vi "HexDAQ.vi"() -> ()   [LabVIEW 2020]
doc: "This is the main VI for the HexDAQ project. Contains the front panel controls steers the entire data taking, logging and display."
uses:
  input_params.ctl
  refs_front_panel.ctl
  <extravilib>/ChannelInstances/Tag-a[.](c(a[.](stamp),a[.](dbl)))/Read With Abort.vi
  <extravilib>/ChannelInstances/Tag-bool/Read With Abort.vi
  <extravilib>/ChannelInstances/Tag-t'input_params.ctl'/Write With Abort.vi
  <extravilib>/ChannelInstances/Tag-str/Write With Abort.vi
  <extravilib>/ChannelInstances/Tag-bool/Write With Abort.vi
  <extravilib>/ChannelInstances/Tag-t'data_env.ctl'/Instantiate.vi
  <extravilib>/ChannelInstances/Tag-t'input_params.ctl'/Instantiate.vi
  <extravilib>/ChannelInstances/Tag-str/Instantiate.vi
  <extravilib>/ChannelInstances/Tag-a[.](c(a[.](stamp),a[.](dbl)))/Instantiate.vi
  <extravilib>/ChannelInstances/Tag-bool/Instantiate.vi
  <extravilib>/ChannelInstances/Tag-a[.](c(a[.](stamp),a[.](dbl)))/EndpointRead.vi
  <extravilib>/ChannelInstances/Tag-bool/EndpointRead.vi
  <extravilib>/ChannelInstances/Tag-t'input_params.ctl'/Endpoint.vi
  <extravilib>/ChannelInstances/Tag-str/Endpoint.vi
  <extravilib>/ChannelInstances/Tag-bool/Endpoint.vi
  <extravilib>/ChannelInstances/Tag-bool.lvlib
  <extravilib>/ChannelInstances/Tag-a[.](c(a[.](stamp),a[.](dbl))).lvlib
  <extravilib>/ChannelInstances/Tag-str.lvlib
  user32.dll
  <extravilib>/ChannelInstances/Tag-t'input_params.ctl'.lvlib
panel:
  in  "Annealing (min)":string
  in  "Fluence (neq)":string
  in  "Temperature (deg C)":string
  in  "Measure\nevery n-th*":dbl=1.0
  out "Switchboard enable":bool=TRUE
  in  "HexPlot binary path":path=path "C:/Users/calice/Desktop/ProbeStation/HGCAL_sensor_tests-CALICE_6in_256ch/bin/HexPlot.exe"
  in  "Source device":T1(ring)=enum."Source_6487"
  in  "LCR device":enum16{"LCR_E4980", "AGILENT_4263X"}(ring)
  in  "Mask pad above (uA)":dbl=5.0
  in  "Mask pads":string
  in  "Source interlock?":bool=TRUE
  out "Missing current [%]\n(Sum cells - tot)/tot":dbl format="%#.0f"
  in  "Abort 3":bool
  in  "Polarity: switch only affects contact test":enum32{"Radio Selection 1", "Radio Selection 2"}(radio)
  in  "CV Switch Delay (s)":dbl=0.3
  in  "IV Switch Delay (s)":dbl=0.3
  in  "CV voltage file":path=path "C:/Users/calice/Desktop/ProbeStation/SensorTest_CALICE_6in_256ch/HGCAL_sensor_tests-CALICE_6in_256ch/config/voltagesCV6Inch256.txt"
  in  "IV voltage file":path=path "C:/Users/calice/Desktop/ProbeStation/SensorTest_CALICE_6in_256ch/HGCAL_sensor_tests-CALICE_6in_256ch/config/voltagesIV.txt"
  in  "Abort 2":bool
  in  "Total curr/vlt \nevery x pads":i32=10
  in  "Disable Switchcard":bool
  in  "Comments (saved in data file)":string
  in  "Needle?":bool
  out "Total current":cluster{i32[], dbl[]}[](graph) caption="XY Graph"
  in  "CV voltage delay (s)":dbl=20.0
  in  "Sensor type":T2(ring)=enum."CALICE_6in_256ch"
  in  "Custom pads":string
  in  "Measurement type":T3(ring)=enum."Debug"
  in  "Hex pad numbers?":bool=TRUE
  in  "?":refnum<k7>(container)
  in  "Custom\nvoltages IV":string
  out "Single channel IV/CV curve":cluster{"X array":dbl[], "Y array":dbl[]}[](graph) caption="XY Graph"
  in  "Repeat":i32=1
  in  "LCR signal voltage (V)":dbl=0.501
  in  "LCR signal frequenzy (kHz)":dbl=2.0 format="%#_13g"
  in  "Sampling number":i32=3
  in  "Picoammeter device":T4(ring)=enum."Keithley6487"
  in  "Take environmental sensor data from":T5(ring)=enum."Probecard"
  out "Environmental data":cluster{timestamp[], dbl[]}[](graph)
  out "Elapsed time":dbl format="%<%H:%M:%S>t"
  out "Estimated remaining time":dbl format="%<%H:%M:%S>t"
  out "Channel values":cluster{i32[], dbl[]}[](graph) caption="XY Graph"
  out "Current channel":dbl format="%#_13g"
  out "Current source voltage (V)":dbl format="%#_13g"
  in  "Abort":bool
  in  "END DAQ":bool
  in  "START DAQ":bool
  in  "Custom\nvoltages CV":string
  in  "Data storage location:":path=path "D:/ProbeStationData"
  in  "Plot after execution?":bool=TRUE
  in  "Voltage limit (V)":dbl=100.0
  in  "Compliance  level (uA)":dbl=2000.0
  in  "VISA resource name LCR":refnum<visa-resource-name>="GPIB0::17::INSTR"
  in  "VISA resource name DMM":refnum<visa-resource-name>="GPIB0::22::INSTR"
  in  "VISA resource name source":refnum<visa-resource-name>="GPIB0::22::INSTR"
  in  "IV voltage delay (s)":dbl=5.0
  in  "Display/needle\nchannel":i32=199
  in  "Identifier (eg. wafer number)":string="Debug"
  # "HexDAQ (v1.8)\nThe LabVIEW program for HGCAL sensor tests\nPlease use issue tracker for feedback and bug reports:\nhttps://gitlab.cern.ch/CLICdp/HGCAL/HGCAL_sensor_tests"
  # "Measurement settings"
  # "Bookkeeping settings"
  # "Both used to determine  the folder and file names"
  # "Timing settings"
  # "(Opt) ID postfixes, leave empty when not wanted"
  # "*not applied for IV measurements"
  # "Device settings"
  # "Debug settings"
  # "VISA settings"
  # "Data storage and visualisation (HexPlot) settings"
  # "Ctrl+H for full display"
  # "p-type sensor"
  # "n-type sensor"
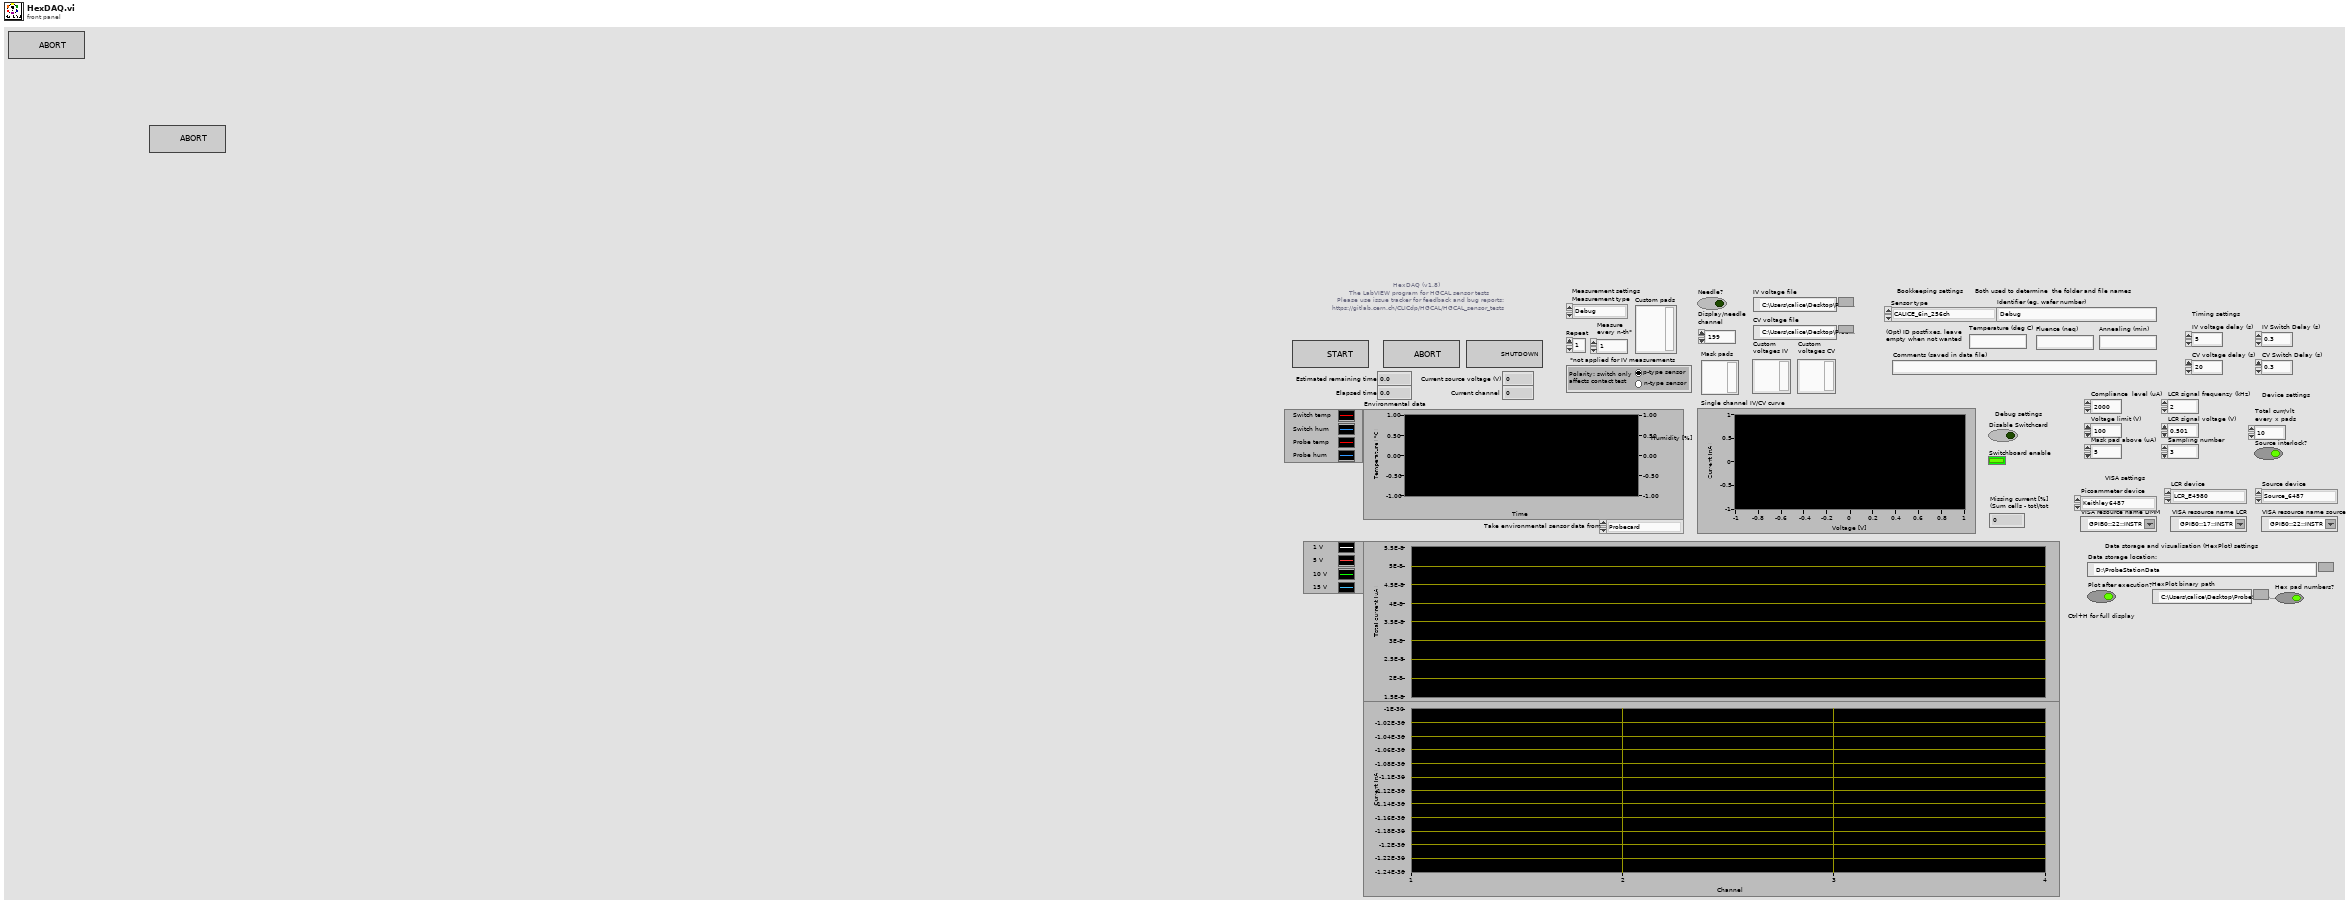
[diagram p1: front panel]
types:
  T1 = enum16{"Source_2410", "Source_6487", "Source_2470"}
  T2 = enum16{"HPK_6in_135ch", "HPK_8in_271ch", "IFX_8in_256ch", "Diode", "HPK_6in_239ch", "Full_Matrix", "HPK_8in_271ch_full", "LumiCal", "HPK_8in_444ch", "HPK_8in_198ch_2019", "HPK_8in_MGW_LD_full", "HPK_8in_MGW_LD_a_type_top", "HPK_8in_MGW_LD_a_type_bottom", "HPK_8in_MGW_LD_b_type_left", "HPK_8in_MGW_LD_b_type_right", "HPK_8in_MGW_LD_c_type_left", "HPK_8in_MGW_LD_c_type_right", "HPK_8in_MGW_HD_full", "HPK_8in_MGW_HD_a_type_top", "HPK_8in_MGW_HD_a_type_bottom", "HPK_8in_MGW_HD_b_type_left", "HPK_8in_MGW_HD_b_type_right", "HPK_8in_MGW_HD_c_type_left", "HPK_8in_MGW_HD_c_type_right", "CALICE_6in_256ch"}
  T3 = enum16{"IV", "CV", "Debug", "Test_contact", "IV+CV"}
  T4 = enum16{"Keithley2001", "Keithley2450", "Keithley2410", "Keithley6485", "Keithley6487", "Keithley6517"}
  T5 = enum16{"Sensirion sht1x/7x", "Switch Matrix", "Probecard"}
  T6 = typedef "refs_front_panel.ctl" = cluster{"Current voltage (V)":refnum<vi>, "Elapsed time":refnum<vi>, "Current channel":refnum<vi>, "Abort":refnum<vi>, "Estimated remaining time":refnum<vi>, "Channel values XYGraph":refnum<vi>, "Single channel XYGraph":refnum<vi>, "Total current XYGraph":refnum<vi>, "Missing\ncurrent [%]":refnum<vi>}
  T7 = typedef "input_params.ctl" = cluster{"Measurement type":enum16{"IV", "CV", "Debug", "Test_contact"}, "Sensor type":enum16{"HPK_6in_135ch", "HPK_8in_271ch", "IFX_8in_256ch", "Diode", "HPK_6in_239ch", "Full_Matrix", "HPK_8in_271ch_full", "LumiCal", "HPK_8in_444ch", "HPK_8in_198ch_2019", "HPK_8in_MGW_LD_full", "HPK_8in_MGW_LD_a_type_top", "HPK_8in_MGW_LD_a_type_bottom", "HPK_8in_MGW_LD_b_type_left", "HPK_8in_MGW_LD_b_type_right", "HPK_8in_MGW_LD_c_type_left", "HPK_8in_MGW_LD_c_type_right", "HPK_8in_MGW_HD_full", "HPK_8in_MGW_HD_a_type_top", "HPK_8in_MGW_HD_a_type_bottom", "HPK_8in_MGW_HD_b_type_left", "HPK_8in_MGW_HD_b_type_right", "HPK_8in_MGW_HD_c_type_left", "HPK_8in_MGW_HD_c_type_right", "CALICE_6in_256ch"}, "Identifier":string, "Open after execution?":bool, "Plot after execution?":bool, "Display channel":i32, "Voltage Delay (s)":dbl, "Switch Delay (s)":dbl, "VISA resource name source":refnum<visa-resource-name>, "VISA resource name DMM":refnum<visa-resource-name>, "VISA resource name LCR":refnum<visa-resource-name>, "Compliance  Level (A)":dbl, "Voltage Limit (V)":dbl, "Data storage location":string, "Scan voltages":string, "Use source as DMM?":bool, "LCR signal frequenzy (Hz)":dbl, "DMM device":enum16{"Keithley2001", "Keithley2450", "Keithley2410", "Keithley6485", "Keithley6487", "Keithley6517"}, "Sampling number":i32, "Use env. sensors on":enum16{"Sensirion sht1x/7x", "Switch Matrix", "Probecard"}, "Switchboard Handle":u32, "Use Switchboard":bool, "LCR signal voltage (V)":dbl, "Repeat":i32, "Scan voltages IV":string, "Scan voltages CV":string, "Hex pad numbers?":bool, "Set measurement type":enum16{"IV", "CV", "Debug", "Test_contact", "IV+CV"}, "Custom pad scan":string, "IV voltage Delay (s)":dbl, "CV voltage Delay (s)":dbl, "Needle measurement?":bool, "Comments":string, "LCR signal frequenzy (kHz)":dbl, "Compliance  Level (uA)":dbl, "Open Correction Array":dbl[][], "Current set voltage":dbl, "Last set voltage":dbl, "Current channel":i32, "Last OpenCorrection index":i32, "Total curr/vltg every x steps":i32, "Current channel iteration":i32, "No CV corrections":bool, "Mapfile":string, "Corrfile":string, "IV voltage file":path, "CV voltage file":path, "IV Switch Delay (s)":dbl, "CV Switch Delay (s)":dbl, "Invert polarity":bool, "Set debug dirs":bool, "Is n on p":bool, "Source interlock?":bool, "Voltage file used?":bool, "Pad mask":string, "Mask pad above (uA)":dbl, "LCR device":enum16{"LCR_E4980", "AGILENT_4263X"}, "Source device":enum16{"Source_2410", "Source_6487", "Source_2470"}, "HexPlot binary path":string, "PadReductionFactor":dbl, "Temperature degC":string, "Fluence [neq]":string, "Annealing [min]":string}
  T8 = typedef "Tag-t'input_params.ctl'.lvlib/))Channel.ctl" = refnum<queue>
  T9 = typedef "Tag-str.lvlib/))Channel.ctl" = refnum<queue>
  T10 = typedef "data_dynamic.ctl" = cluster{"Output file":path, "Y-label text":string, "Current set voltage":dbl, "Set voltage column":dbl[], "Pad number column":dbl[], "Data  column":dbl[], "Number of voltages":i32, "Compliance current (A)":dbl, "Geofile":string, "Peak voltage":dbl, "Hex PDF file":string, "Voltage array":dbl[], "Total current column":dbl[], "Timestamp column":dbl[], "Data name":string, "Data unit":string, "2nd data column":dbl[], "2nd data name":string, "2nd data unit":string, "3rd data column":dbl[], "4th data column":dbl[], "3rd data name":string, "3rd data unit":string, "4th data name":string, "4th data unit":string, "Actual voltage column":dbl[], "2nd Y-label text":string, "Single channel plot":path, "Temperature column":dbl[], "Humidity column":dbl[], "Channel switch array":i32[], "1st single plot name":string, "2nd single plot name":string, "All channels plot":path, "HexPlot command":string, "Custom channel array":i32[], "Data  error column":dbl[], "2nd data  error column":dbl[], "3rd data error column":dbl[], "4th data  error column":dbl[], "Total current plot":path, "5th data column":dbl[], "5th data  error column":dbl[], "6th data column":dbl[], "6th data  error column":dbl[], "5th data name":string, "5th data unit":string, "6th data name":string, "6th data unit":string, "HexPlot matrix command":string, "HexPlot analysis command":string}
  T11 = typedef "Tag-bool.lvlib/))Channel.ctl" = refnum<queue>
  T12 = typedef "Tag-a[.](c(a[.](stamp),a[.](dbl))).lvlib/))Channel.ctl" = refnum<queue>
  T13 = typedef "Tag-t'data_env.ctl'.lvlib/))Channel.ctl" = refnum<queue>
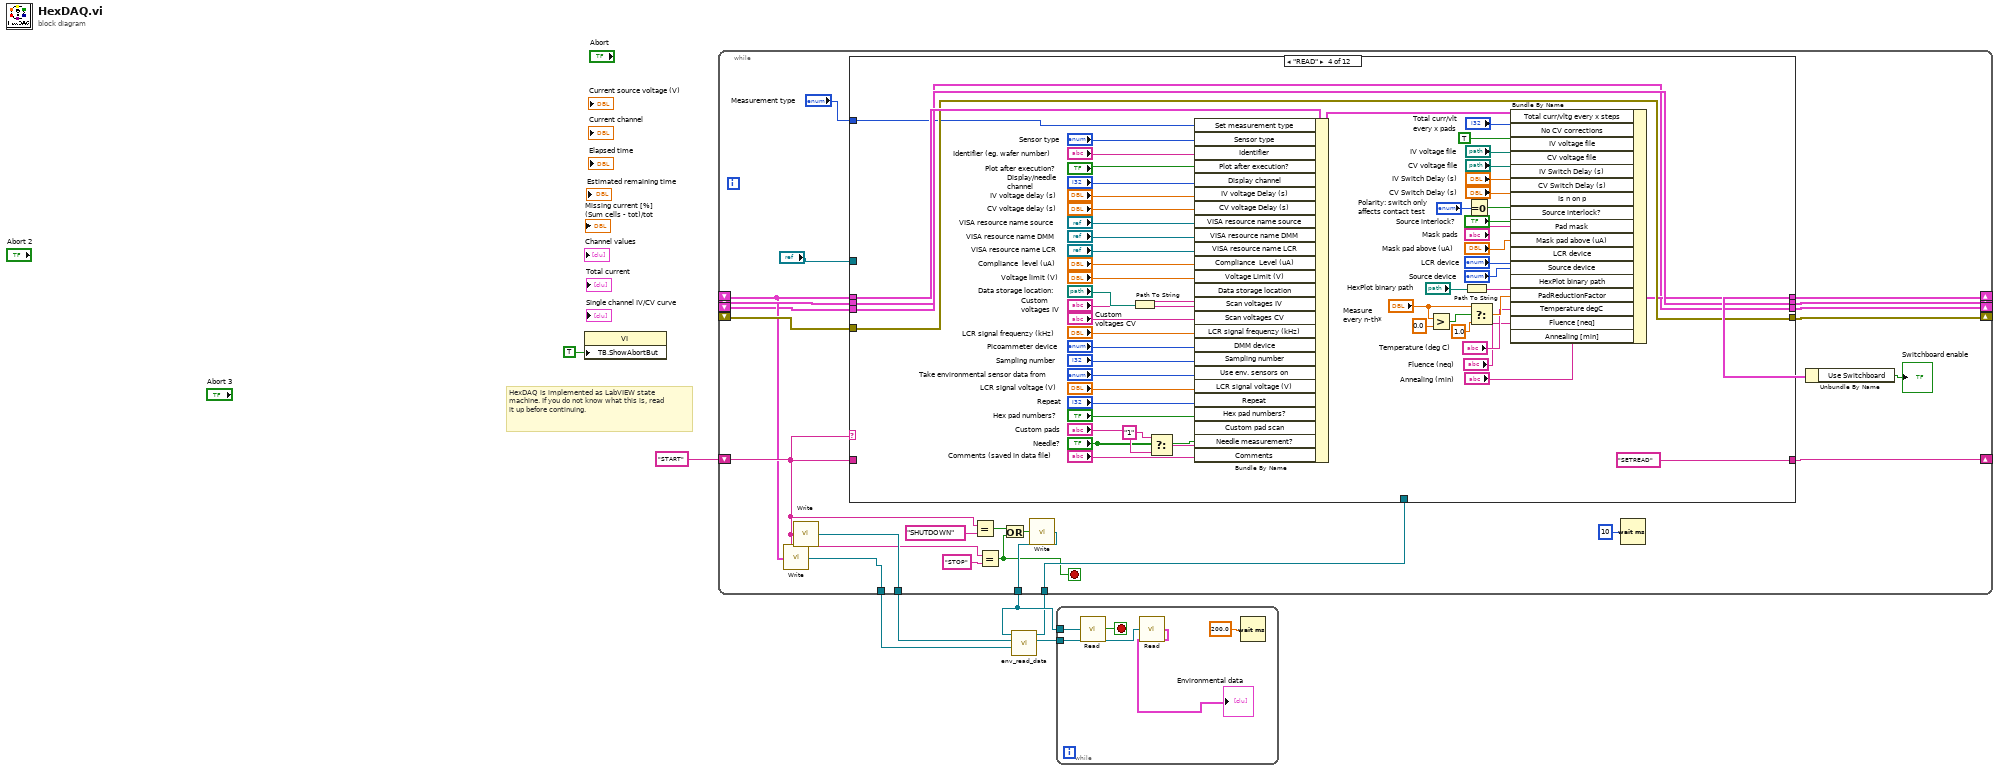
[diagram p0: block diagram]
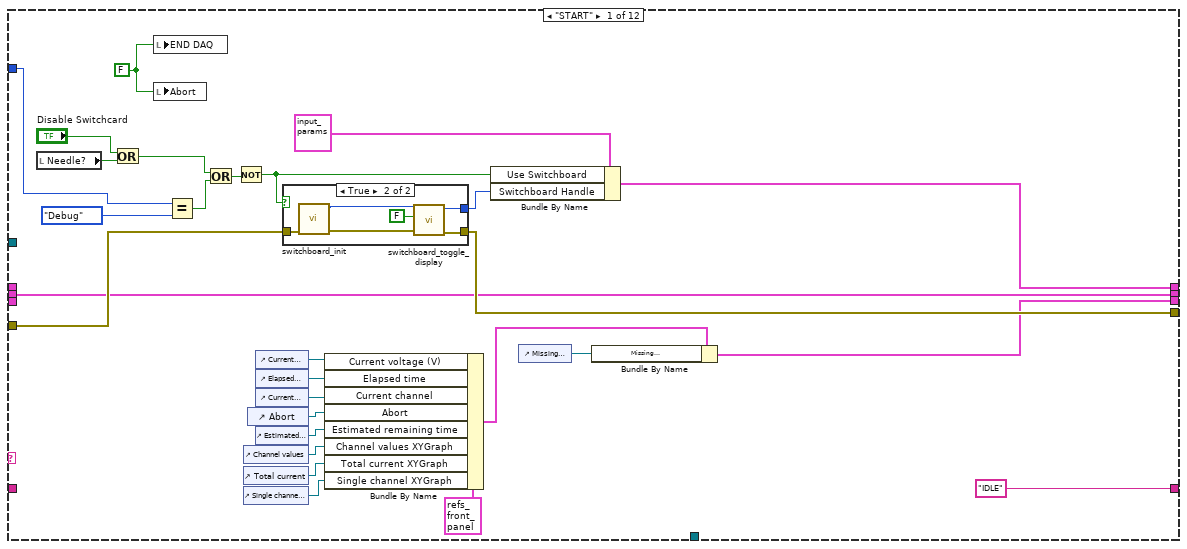
[diagram p2: hidden frame]
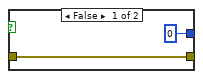
[diagram p3: hidden frame]
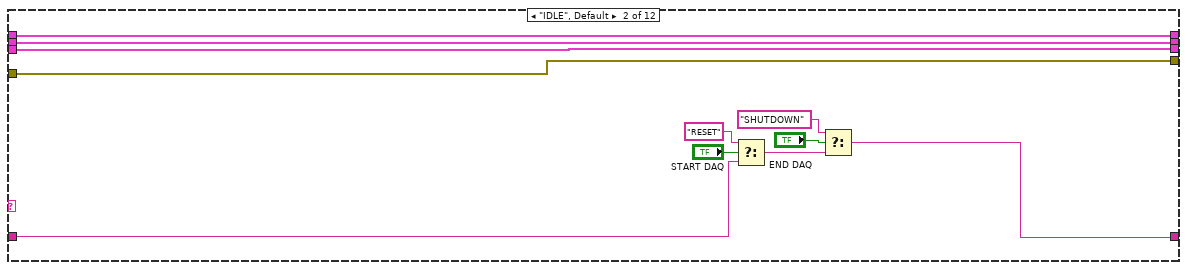
[diagram p4: hidden frame]
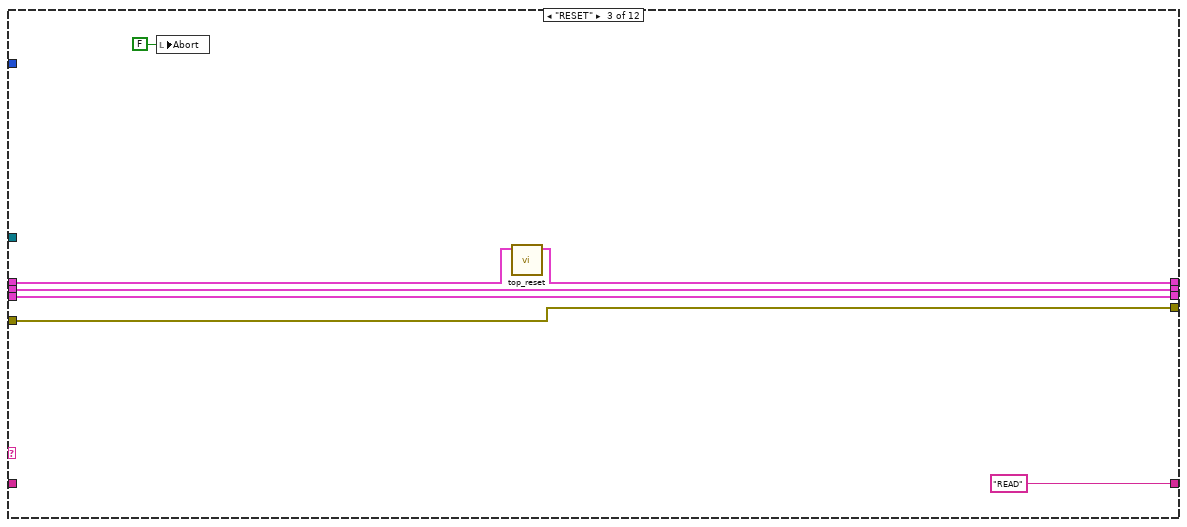
[diagram p5: hidden frame]
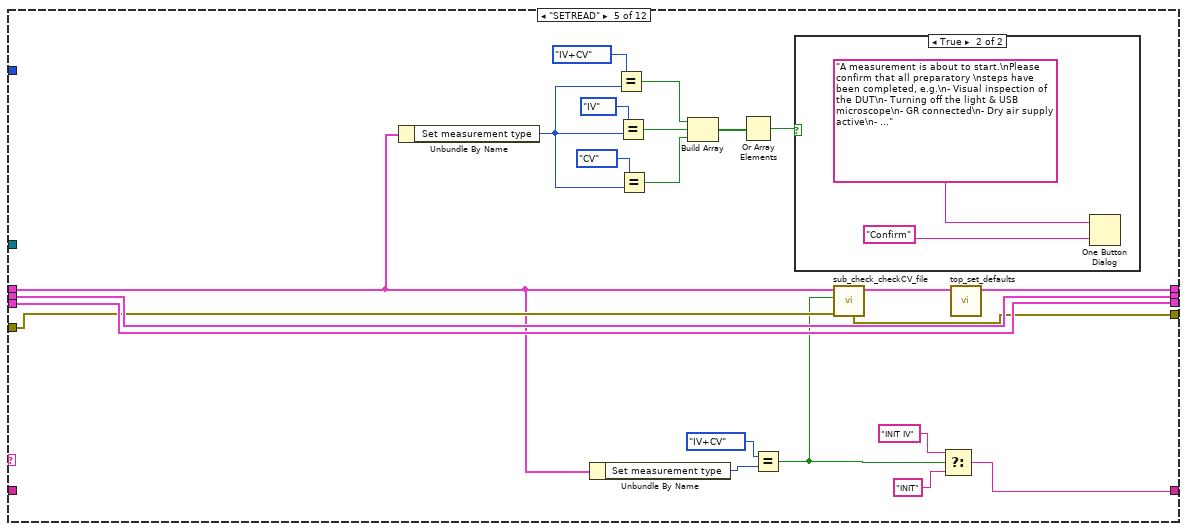
[diagram p6: hidden frame]
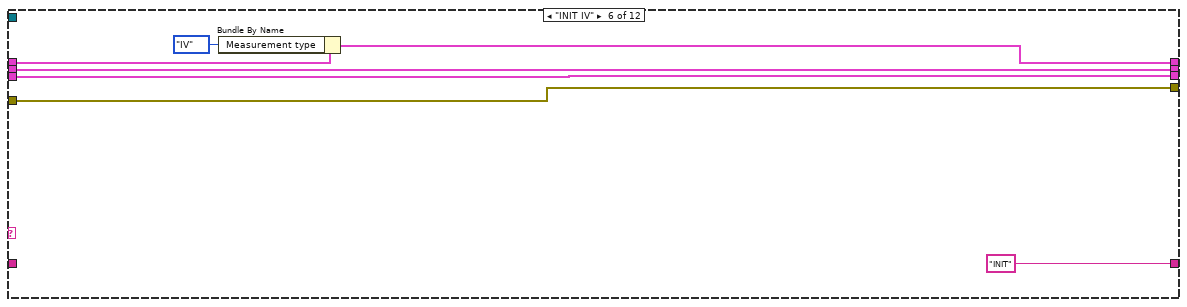
[diagram p8: hidden frame]
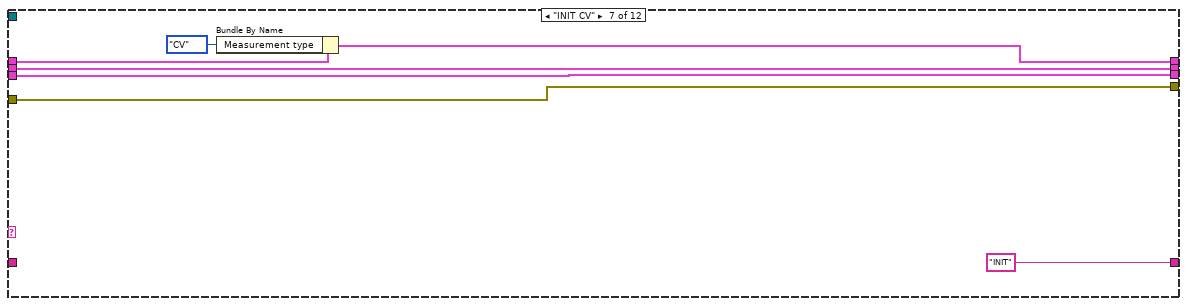
[diagram p9: hidden frame]
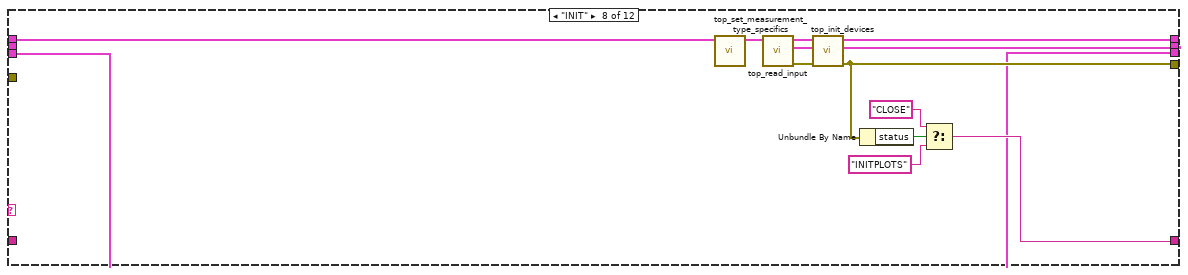
[diagram p10: hidden frame]
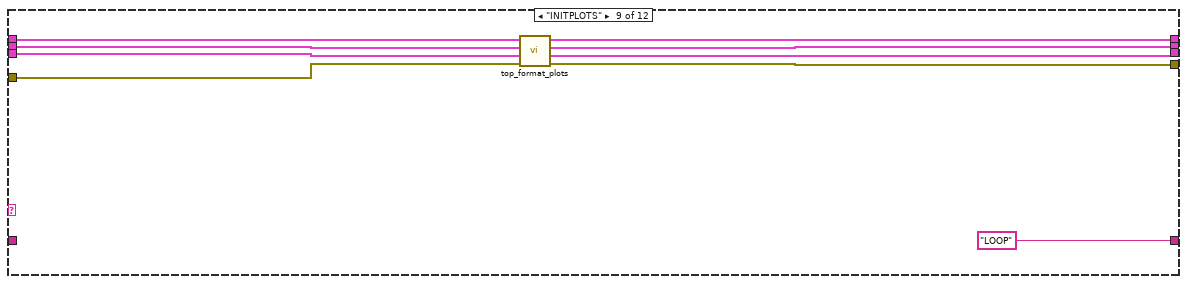
[diagram p11: hidden frame]
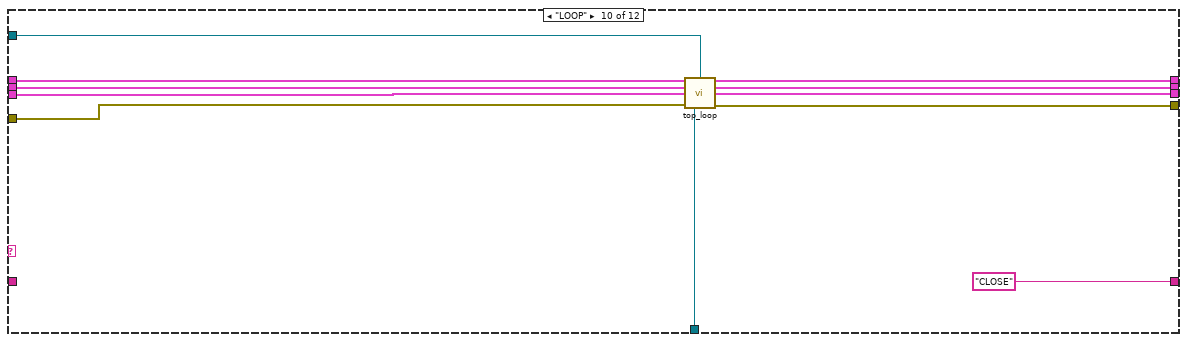
[diagram p12: hidden frame]
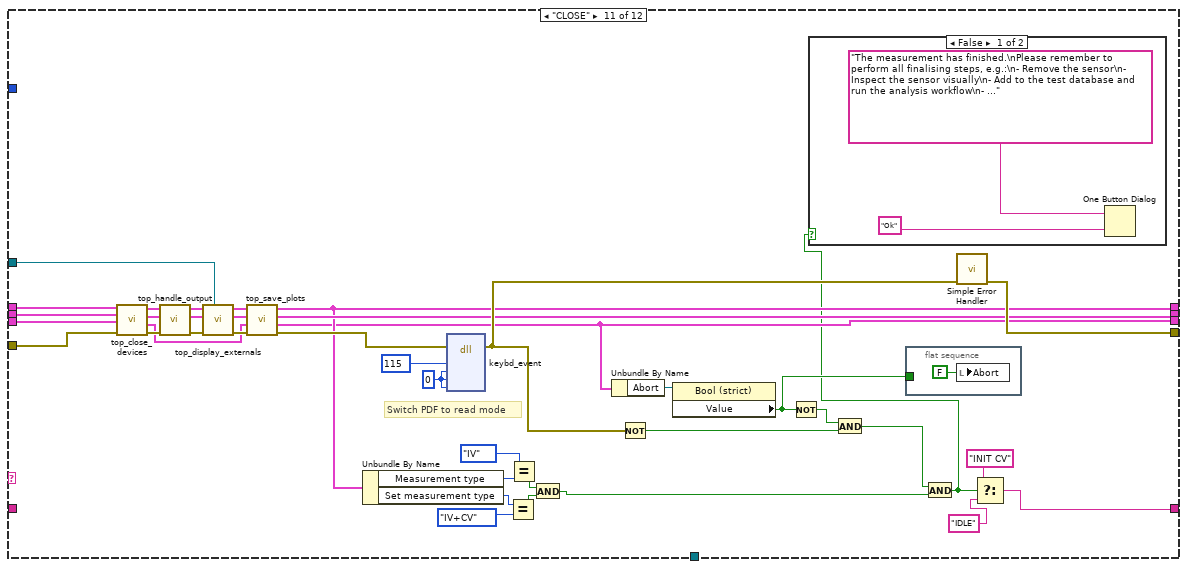
[diagram p13: hidden frame]
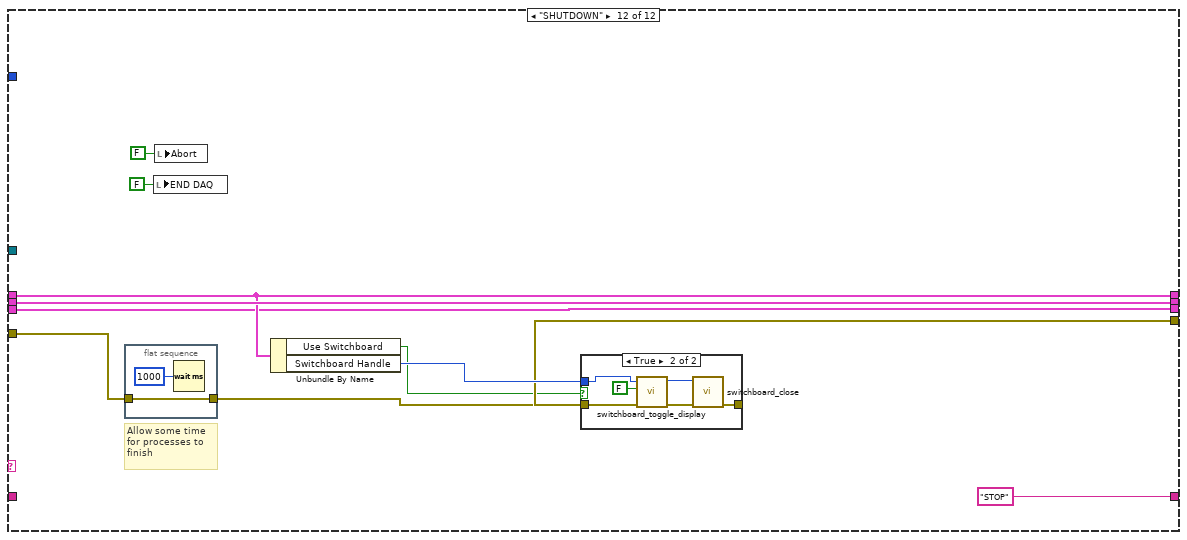
[diagram p15: hidden frame]
diagram:
  # "HexDAQ is implemented as LabVIEW state machine. If you do not know what this is, read it up before continuing."
  n1 = property class="VI"("TB.ShowAbortBut"=TRUE ("Tool Bar:Show Abort Button")) -> ()  [unwired: 2 in, 2 out]
  n2 = while {
    shift-right: [w30] -> _
    shift-left: "START" -> [w19]
    shift-right: [w26] -> _
    shift-left: _ -> [w24]
    shift-right: [w27] -> _
    shift-left: _ -> [w25]
    shift-right: [w9] -> _
    shift-left: _ -> [w15]
    tunnel: [w23] -> w5
    tunnel: w1 -> [w22]
    tunnel: [w21] -> w3
    tunnel: [w11] -> w2
    shift-right: [w13] -> _
    shift-left: _ -> [w12]
    stop <- w16 stop-if-true
    n3 = call <extravilib>:"Write.vi"("element"=w15) -> ("channel"=w11:T8)  [unwired: 1 out]
    n4 = call <extravilib>:"Write.vi"("element"=w19) -> ("channel"=w21:T9)  [unwired: 1 out]
    n5 = case shown="\"READ\"" w19 {
      tunnel: w19 -> [_ w77 _ _ _ _ _ _ _ _ _ _]
      tunnel: ["IDLE" ("t") w74 "READ" ("t") "SETREAD" ("t") w160 "INIT" ("t") "INIT" ("t") w184 "LOOP" ("t") "CLOSE" ("t") w232 "STOP" ("t")] -> w30
      tunnel: [w52 w70 w79 w116 w158 w170 w177 w190 w198 w212 w223 w259] -> w9
      tunnel: [w56 w69 w83 w122 w155 w173 w180 w188 w194 w210 w244 w263] -> w26
      tunnel: [w53 w68 w80 w123 w164 w172 w179 w189 w197 w211 w225 w265] -> w27
      tunnel: w15 -> [_ w70 w78 w124 w152 w171 w178 w182 w201 w207 w246 w259]
      tunnel: w25 -> [w53 w68 w80 w123 w164 w172 w179 _ w202 w208 w242 w265]
      tunnel: w24 -> [w57 w69 w83 w122 w156 w173 w180 _ w195 w209 w245 w261]
      tunnel: "?" -> [_ _ _ _ _ _ _ _ _ w203 w243 _]
      tunnel: w22 -> [_ _ _ _ _ _ _ _ _ w206 _ _]
      tunnel: [w39 w67 w82 w114 w157 w167 w174 w183 w196 w205 w222 w258] -> w13
      tunnel: w12 -> [_ w67 w82 w114 w157 w167 w174 w183 w199 w204 w216 w258]
      tunnel: "Measurement type" -> [w31 _ _ w103 _ _ _ _ _ _ _ _]
      frame "START" {
        w40 = FALSE ("Abort")
        n6 = local read "Needle?"() -> (w50:bool)
        n7 = Or(x="Disable Switchcard", y=w50) -> (x .or. y?=w35:bool)
        n8 = local write "END DAQ"(w40) -> ()
        n9 = local write "Abort"(w40) -> ()
        n10 = Equal?(x=w31, y=T3."Debug" ("Measurement type")) -> (x = y?=w34:bool)
        n11 = Or(x=w35, y=w34) -> (x .or. y?=w33:bool)
        n12 = Not(x=w33) -> (.not. x?=w32:bool)
        n13 = control-ref of="Channel values"() -> (w43:refnum<vi>)
        n14 = control-ref of="Total current"() -> (w42:refnum<vi>)
        n15 = control-ref of="Single channel IV/CV curve"() -> (w41:refnum<vi>)
        n16 = control-ref of="Abort"() -> (w45:refnum<vi>)
        n17 = control-ref of="Current source voltage (V)"() -> (w47:refnum<vi>)
        n18 = control-ref of="Elapsed time"() -> (w48:refnum<vi>)
        n19 = control-ref of="Current channel"() -> (w46:refnum<vi>)
        n20 = control-ref of="Estimated remaining time"() -> (w44:refnum<vi>)
        n21 = case shown="True" w32 {
          tunnel: w57 -> [w60 w66]
          tunnel: [w60 w65] -> w56
          tunnel: [u32 0 ("Handle") w63] -> w55
          frame False {
          }
          frame True {
            n22 = call <instrlib>:"switchboard_init.vi"("error in"=w66) -> ("error out"=w62:errorcluster, "Handle"=w61:u32)  [unwired: 9 in]
            n23 = call <instrlib>:"switchboard_toggle_display.vi"("error in"=w62, "On/Off"=FALSE, "Handle"=w61) -> ("error out"=w65:errorcluster, "Handle out"=w63:u32)  [unwired: 7 in]
          }
        }
        n24 = Bundle By Name(cluster=T6 {"Current voltage (V)"=refnum, "Elapsed time"=refnum, "Current channel"=refnum, "Abort"=refnum, "Estimated remaining time"=refnum, "Channel values XYGraph"=refnum, "Single channel XYGraph"=refnum, "Total current XYGraph"=refnum, "Missing\ncurrent [%]"=refnum} ("Cluster"), "Current voltage (V)"=w47, "Elapsed time"=w48, "Current channel"=w46, "Abort"=w45, "Estimated remaining time"=w44, "Channel values XYGraph"=w43, "Total current XYGraph"=w42, "Single channel XYGraph"=w41) -> (w38:T6)
        n25 = Bundle By Name(cluster=T7 {"Measurement type"=enum."Debug", "Sensor type"=enum."HPK_6in_135ch", "Identifier"="test.txt", "Open after execution?"=FALSE, "Plot after execution?"=FALSE, "Display channel"=0, "Voltage Delay (s)"=0.5, "Switch Delay (s)"=0.01, "VISA resource name source"="", "VISA resource name DMM"="", "VISA resource name LCR"="", "Compliance  Level (A)"=10.0, "Voltage Limit (V)"=1000.0, "Data storage location"="", "Scan voltages"="", "Use source as DMM?"=FALSE, "LCR signal frequenzy (Hz)"=10.0, "DMM device"=enum."Keithley2001", "Sampling number"=1, "Use env. sensors on"=enum."Sensirion sht1x/7x", "Switchboard Handle"=0, "Use Switchboard"=FALSE, "LCR signal voltage (V)"=10000.0, "Repeat"=1, "Scan voltages IV"="", "Scan voltages CV"="", "Hex pad numbers?"=FALSE, "Set measurement type"=enum."Debug", "Custom pad scan"="", "IV voltage Delay (s)"=0.5, "CV voltage Delay (s)"=0.5, "Needle measurement?"=FALSE, "Comments"="test.txt", "LCR signal frequenzy (kHz)"=10.0, "Compliance  Level (uA)"=10.0, "Open Correction Array"=array2304x3[6912 elements], "Current set voltage"=0.0, "Last set voltage"=0.0, "Current channel"=0, "Last OpenCorrection index"=-1, "Total curr/vltg every x steps"=10, "Current channel iteration"=0, "No CV corrections"=FALSE, "Mapfile"="", "Corrfile"="", "IV voltage file"=path "", "CV voltage file"=path "", "IV Switch Delay (s)"=0.01, "CV Switch Delay (s)"=0.01, "Invert polarity"=FALSE, "Set debug dirs"=FALSE, "Is n on p"=FALSE, "Source interlock?"=TRUE, "Voltage file used?"=FALSE, "Pad mask"="", "Mask pad above (uA)"=1.0, "LCR device"=enum."LCR_E4980", "Source device"=enum."Source_2410", "HexPlot binary path"="", "PadReductionFactor"=1.0, "Temperature degC"="", "Fluence [neq]"="", "Annealing [min]"=""} ("Input parameters"), "Use Switchboard"=w32, "Switchboard Handle"=w55) -> (w52:T7)
        n26 = control-ref of="Missing current [%]\n(Sum cells - tot)/tot"() -> (w37:refnum<vi>)
        n27 = Bundle By Name(cluster=w38, "Missing\ncurrent [%]"=w37) -> (w39:T6)
      }
      frame "IDLE", Default {
        n28 = Select(t="RESET", s="START DAQ", f=w77) -> (s? t:f=w75:string)
        n29 = Select(t="SHUTDOWN", s="END DAQ", f=w75) -> (s? t:f=w74:string)
      }
      frame "RESET" {
        n30 = local write "Abort"(FALSE ("Abort")) -> ()
        n31 = call "top_reset.vi"("Input parameters"=w78) -> ("New input parameters"=w79:T7)  [unwired: 10 in]
      }
      frame "READ" {
        n32 = Path To String(path="Data storage location:") -> (string=w127:string)
        n33 = Select(t="1", s="Needle?", f="Custom pads") -> (s? t:f=w100:string)
        n34 = Bundle By Name(cluster=w124, "Set measurement type"=w103, "Sensor type"="Sensor type", "Identifier"="Identifier (eg. wafer number)", "Plot after execution?"="Plot after execution?", "Display channel"="Display/needle\nchannel", "IV voltage Delay (s)"="IV voltage delay (s)", "CV voltage Delay (s)"="CV voltage delay (s)", "VISA resource name source"="VISA resource name source", "VISA resource name DMM"="VISA resource name DMM", "VISA resource name LCR"="VISA resource name LCR", "Compliance  Level (uA)"="Compliance  level (uA)", "Voltage Limit (V)"="Voltage limit (V)", "Data storage location"=w127, "Scan voltages IV"="Custom\nvoltages IV", "Scan voltages CV"="Custom\nvoltages CV", "LCR signal frequenzy (kHz)"="LCR signal frequenzy (kHz)", "DMM device"="Picoammeter device", "Sampling number"="Sampling number", "Use env. sensors on"="Take environmental sensor data from", "LCR signal voltage (V)"="LCR signal voltage (V)", "Repeat"="Repeat", "Hex pad numbers?"="Hex pad numbers?", "Custom pad scan"=w100, "Needle measurement?"="Needle?", "Comments"="Comments (saved in data file)") -> (w102:T7)
        n35 = Greater?(x="Measure\nevery n-th*", y=0.0) -> (0:w90:bool)
        n36 = Path To String(path="HexPlot binary path") -> (string=w104:string)
        n37 = Equal To 0?(x="Polarity: switch only affects contact test") -> (x = 0?=w95:bool)
        n38 = Select(t="Measure\nevery n-th*", s=w90, f=1.0) -> (s? t:f=w93:dbl)
        n39 = Bundle By Name(cluster=w102, "Total curr/vltg every x steps"="Total curr/vlt \nevery x pads", "No CV corrections"=TRUE, "IV voltage file"="IV voltage file", "CV voltage file"="CV voltage file", "IV Switch Delay (s)"="IV Switch Delay (s)", "CV Switch Delay (s)"="CV Switch Delay (s)", "Is n on p"=w95, "Source interlock?"="Source interlock?", "Pad mask"="Mask pads", "Mask pad above (uA)"="Mask pad above (uA)", "LCR device"="LCR device", "Source device"="Source device", "HexPlot binary path"=w104, "PadReductionFactor"=w93, "Temperature degC"="Temperature (deg C)", "Fluence [neq]"="Fluence (neq)", "Annealing [min]"="Annealing (min)") -> (w116:T7)
      }
      frame "SETREAD" {
        n40 = Unbundle By Name(w152) -> ("Set measurement type"=w150:T3)
        n41 = Unbundle By Name(w152) -> ("Set measurement type"=w159:T3)
        n42 = Equal?(x=T3."IV+CV" ("Measurement type"), y=w150) -> (x = y?=w147:bool)
        n43 = Equal?(x=T3."IV" ("Measurement type"), y=w150) -> (x = y?=w146:bool)
        n44 = Equal?(x=T3."CV" ("Measurement type"), y=w150) -> (x = y?=w145:bool)
        n45 = Build Array(w147, w146, w145) -> (w144:bool[])
        n46 = Or Array Elements(Boolean array=w144) -> (logical OR=w143:bool)
        n47 = Equal?(x=T3."IV+CV" ("Measurement type"), y=w159) -> (x = y?=w153:bool)
        n48 = case shown="True" w143 {
          frame False {
          }
          frame True {
            n49 = One Button Dialog(message="A measurement is about to start.\nPlease confirm that all preparatory \nsteps have been completed, e.g.\n- Visual inspection of the DUT\n- Turning off the light & USB microscope\n- GR connected\n- Dry air supply active\n- ...", button name ("OK")="Confirm") -> ()  [unwired: 1 out]
          }
        }
        n50 = call "sub_check_checkCV_file.vi"("error in"=w156, "Check CVPath"=w153, "Input parameters"=w152) -> ("error out"=w155:errorcluster, "Input parameters out"=w154:T7)  [unwired: 5 in]
        n51 = Select(t="INIT IV", s=w153, f="INIT" ("t")) -> (s? t:f=w160:string)
        n52 = call "top_set_defaults.vi"("Input parameters"=w154) -> ("Input parameters out"=w158:T7)  [unwired: 10 in]
      }
      frame "INIT IV" {
        n53 = Bundle By Name(cluster=w171, "Measurement type"=enum16{"IV", "CV", "Debug", "Test_contact"}."IV") -> (w170:T7)
      }
      frame "INIT CV" {
        n54 = Bundle By Name(cluster=w178, "Measurement type"=enum16{"IV", "CV", "Debug", "Test_contact"}."CV") -> (w177:T7)
      }
      frame "INIT" {
        n55 = call "top_set_measurement_type_specifics.vi"("Input parameters"=w182) -> ("Input parameters out"=w181:T7)  [unwired: 10 in]
        n56 = call "top_read_input.vi"("Input parameters"=w181) -> ("error out"=w192:errorcluster, "Dynamic data"=w191:T10, "Input parameters"=w193:T7)  [unwired: 8 in]
        n57 = call "top_init_devices.vi"("error in (no error)"=w192, "Dynamic data"=w191, "Input parameters"=w193) -> ("error out"=w188:errorcluster, "Dynamic data"=w189:T10, "Input parameters"=w190:T7)  [unwired: 6 in]
        n58 = Unbundle By Name(w188) -> ("status"=w187:bool)
        n59 = Select(t="CLOSE", s=w187, f="INITPLOTS" ("t")) -> (s? t:f=w184:string)
      }
      frame "INITPLOTS" {
        n60 = call "top_format_plots.vi"("error in"=w195, "Front panel refs"=w199, "Dynamic data"=w202, "Input parameters"=w201) -> ("error out"=w194:errorcluster, "Front panel refs out"=w196:T6, "Dynamic data out"=w197:T10, "Input parameters out"=w198:T7)  [unwired: 4 in]
      }
      frame "LOOP" {
        n61 = call "top_loop.vi"("Input parameters"=w207, 2:w203, "Dynamic data"=w208, "Front_panel_refs"=w204, "error in (no error)"=w209, "Environmental data"=w206) -> ("Input parameters out"=w212:T7, "Dynamic data out"=w211:T10, "Front_panel_refs out"=w205:T6, "error out"=w210:errorcluster)  [unwired: 6 in]
      }
      frame "CLOSE" {
        w230 = u8 0 ("bScan")
        # "Switch PDF to read mode"
        n62 = call "top_close_devices.vi"("error in (no error)"=w245, "Front_panel_refs"=w216, "Dynamic data"=w242, "Input parameters"=w246) -> ("error out"=w252:errorcluster, "Front_panel_refs out"=w215:T6, "Dynamic data"=w250:T10, "Input parameters"=w251:T7)  [unwired: 4 in]
        n63 = call "top_handle_output.vi"("error in (no error)"=w252, "Dynamic data"=w250, "Input parameters"=w251) -> ("error out"=w249:errorcluster, "Dynamic data"=w248:T10, "Input parameters"=w247:T7)  [unwired: 6 in]
        n64 = call "top_display_externals.vi"("AcroPDF"=w243, "error in (no error)"=w249, "Dynamic data"=w248, "Input parameters"=w247) -> ("error out"=w241:errorcluster, "Dynamic data"=w226:T10, "Input parameters"=w224:T7)  [unwired: 5 in]
        n65 = call "top_save_plots.vi"("error in"=w241, "Front_panel_refs"=w215, "Dynamic data"=w226, "Input parameters"=w224) -> ("error out"=w228:errorcluster, "Front_panel_refs out"=w222:T6, "Dynamic data out"=w225:T10, "Input parameters out"=w223:T7)  [unwired: 4 in]
        n66 = Unbundle By Name(w223) -> ("Measurement type"=w240:enum16{"IV", "CV", "Debug", "Test_contact"}, "Set measurement type"=w238:T3)
        n67 = dll-call lib="user32.dll" fn="keybd_event"(error in=w228, "bVk"=u8 115 ("Virtual Key"), "bScan"=w230, "dwFlags"=w230, "dwExtraInfo"=w230) -> (error out=w227:errorcluster)  [unwired: 7 in, 1 out]
        n68 = Equal?(x=w238, y=T3."IV+CV") -> (x = y?=w235:bool)
        n69 = Equal?(x=enum16{"IV", "CV", "Debug", "Test_contact"}."IV", y=w240) -> (x = y?=w236:bool)
        n70 = And(x=w236, y=w235) -> (x .and. y?=w218:bool)
        n71 = Unbundle By Name(w222) -> ("Abort"=w221:refnum<vi>)
        n72 = Not(x=w227) -> (.not. x?=w219:bool)
        n73 = property class="Bool (strict)"(reference=w221) -> ("Value"=w231:bool)  [unwired: 1 in, 2 out]
        n74 = Not(x=w231) -> (.not. x?=w220:bool)
        n75 = And(x=w220, y=w219) -> (x .and. y?=w217:bool)
        n76 = flat-sequence {
          tunnel: w231 -> [_]
          frame #0 {
            n77 = local write "Abort"(FALSE ("Abort")) -> ()
          }
        }
        n78 = And(x=w217, y=w218) -> (x .and. y?=w214:bool)
        n79 = case shown="False" w214 {
          frame False {
            n80 = One Button Dialog(message="The measurement has finished.\nPlease remember to perform all finalising steps, e.g.:\n- Remove the sensor\n- Inspect the sensor visually\n- Add to the test database and run the analysis workflow\n- ...", button name ("OK")="Ok") -> ()  [unwired: 1 out]
          }
          frame True {
          }
        }
        n81 = call <vilib>:"Simple Error Handler.vi"("error in (no error)"=w227) -> ("error out"=w244:errorcluster)  [unwired: 4 in, 4 out]
        n82 = Select(t="INIT CV", s=w214, f="IDLE" ("t")) -> (s? t:f=w232:string)
      }
      frame "SHUTDOWN" {
        # "Allow some time\nfor processes to\nfinish"
        n83 = flat-sequence {
          tunnel: w261 -> [w267]
          tunnel: [w267] -> w260
          frame #0 {
            n84 = Wait (ms)(milliseconds to wait=u32 1000) -> ()  [unwired: 1 out]
          }
        }
        n85 = local write "END DAQ"(FALSE ("END DAQ")) -> ()
        n86 = local write "Abort"(FALSE ("Abort")) -> ()
        n87 = Unbundle By Name(w259) -> ("Use Switchboard"=w256:bool, "Switchboard Handle"=w264:u32)
        n88 = case shown="True" w256 {
          tunnel: w260 -> [w269 w273]
          tunnel: [w269 w275] -> w263
          tunnel: w264 -> [_ w272]
          frame False {
          }
          frame True {
            n89 = call <instrlib>:"switchboard_toggle_display.vi"("error in"=w273, "On/Off"=FALSE, "Handle"=w272) -> ("error out"=w270:errorcluster, "Handle out"=w271:u32)  [unwired: 7 in]
            n90 = call <instrlib>:"switchboard_close.vi"("error in"=w270, "Handle"=w271) -> ("error out"=w275:errorcluster)  [unwired: 8 in, 1 out]
          }
        }
      }
    }
    n91 = Equal?(x=w19, y="SHUTDOWN") -> (x = y?=w18:bool)
    n92 = Equal?(x=w19, y="STOP") -> (x = y?=w16:bool)
    n93 = Or(x=w18, y=w16) -> (x .or. y?=w17:bool)
    n94 = call <extravilib>:"Write.vi"("element"=w17) -> ("channel"=w23:T11)  [unwired: 1 out]
    n95 = Wait (ms)(milliseconds to wait=u32 10) -> ()  [unwired: 1 out]
    n96 = Unbundle By Name(w9) -> ("Use Switchboard"=→"Switchboard enable":bool)
  }
  n97 = call "env_read_data.vi"("Input parameters"=w2, "State"=w3, "Stop signal"=w5) -> ("Plot data out"=w4:T12, "channel"=w1:T13)  [unwired: 6 in, 1 out]
  n98 = while {
    tunnel: w5 -> [w279]
    tunnel: w4 -> [w277]
    stop <- w278 stop-if-true
    n99 = call <extravilib>:"Read.vi"("channel"=w279) -> ("element"=w278:bool)  [unwired: 1 in, 1 out]
    n100 = call <extravilib>:"Read.vi"("channel"=w277) -> ("element"=→"Environmental data":cluster{timestamp[], dbl[]}[])  [unwired: 1 in, 1 out]
    n101 = Wait (ms)(milliseconds to wait=sgl 200.0 ("Sample period (s)")) -> ()  [unwired: 1 out]
  }
